vi "Configure Output.vi"(3 "error in (no error)":errorcluster, 4 "Output On":bool, 5 "VISA resource name":refnum<visa-resource-name>) -> (0 "error out":errorcluster, 2 "VISA resource name out":refnum<visa-resource-name>)   [LabVIEW 2019, in "9103Series.lvlib"]
uses:
  <instrlib>/9103Series/9103Series.lvlib
panel:
  out "ok?":string
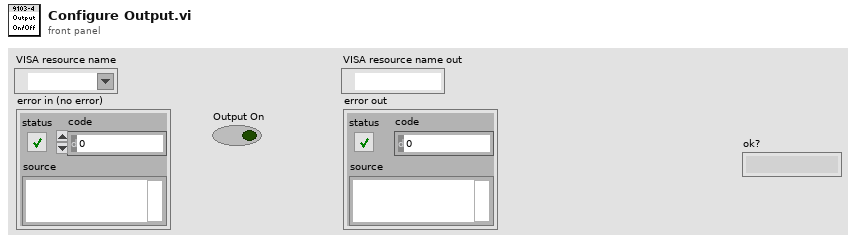
[diagram p1: front panel]
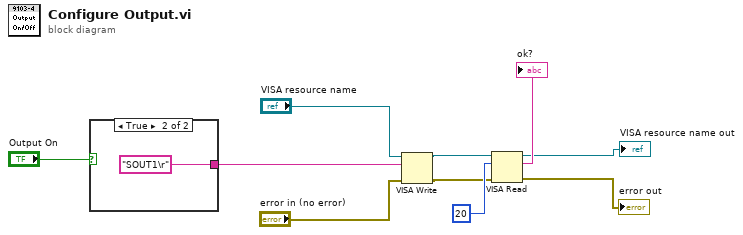
[diagram p0: block diagram]
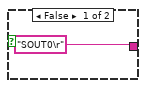
[diagram p2: hidden frame]
diagram:
  n1 = case shown="True" "Output On" {
    tunnel: ["SOUT0\r" ("string") "SOUT1\r" ("string")] -> w8
    frame False {
    }
    frame True {
    }
  }
  n2 = VISA Write(VISA resource name="VISA resource name", write buffer=w8, error in (no error)="error in (no error)") -> (VISA resource name out=w4:refnum<visa-resource-name>, error out=w3:errorcluster)  [unwired: 1 out]
  n3 = VISA Read(VISA resource name=w4, byte count=u32 20, error in (no error)=w3) -> (VISA resource name out=→"VISA resource name out":refnum<visa-resource-name>, read buffer=→"ok?":string, error out=→"error out":errorcluster)  [unwired: 1 out]
